vi "LVDimInterface.release.vi"(5 "error in (no error)":errorcluster) -> (19 "error out":errorcluster)   [LabVIEW 2013, in "LVDimInterface.lvlib"]
doc: "Releases (unlocks) the LVDimInterface after changes. This routine is intended for internal purposes only.\n\nLicense Agreement for this software:\n\nCopyright (C)\nGesellschaft für Schwerionenforschung, GSI\nPlanckstr. 1\n64291 Darmstadt\nGermany\n\nContact: D.Beck@gsi.de \n\nThis program is free software; you can redistribute it and/or modify it under the terms of the GNU General Public License as published by the Free Software Foundation; either version 2 of the license, or (at your option) any later version.\n\nThis program is distributed in the hope that it will be useful, but WITHOUT ANY WARRANTY; without even the implied warranty of MERCHANTABILITY or FITNESS FOR A PARTICULAR PURPOSE. See the GNU General License for more details (http://www.gnu.org).\n\nGesellschaft für Schwerionenforschung, GSI\nPlanckstr. 1, 64291 Darmstadt, Germany\nFor all questions and ideas contact: M.Richter@gsi.de, H.Brand@gsi.de or D.Beck@gsi.de.\nLast update: 17-JUN-2004"
uses:
  LVDimInterface.lvlib
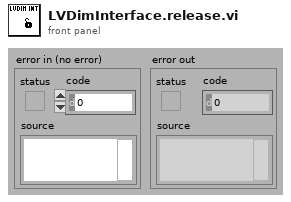
[diagram p1: front panel]
types:
  T1 = enum16{"unknown", "createSemaphore", "destroySemaphore", "getSemaphore"}
  T2 = typedef "Semaphore RefNum" = refnum<k1>
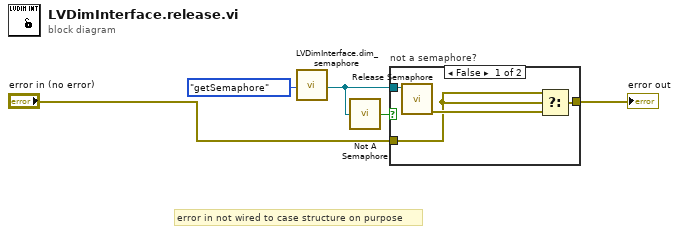
[diagram p0: block diagram]
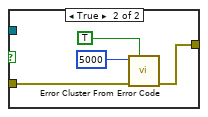
[diagram p2: hidden frame]
diagram:
  # "error in not wired to case structure on purpose"
  n1 = call "LVDimInterface.dim_semaphore.vi"("Action"=T1."getSemaphore") -> ("semaphore"=w2:T2)  [unwired: 18 in]
  n2 = call <vilib>:"Not A Semaphore.vi"("semaphore"=w2) -> ("not a semaphore"=w3:bool)
  n3 = case "not a semaphore?" shown="False" w3 {
    tunnel: [w9 w12] -> w5
    tunnel: "error in (no error)" -> [w7 w13]
    tunnel: w2 -> [w6 _]
    frame False {
      n4 = call <vilib>:"Release Semaphore.vi"("semaphore"=w6) -> ("error out"=w8:errorcluster)  [unwired: 5 in, 1 out]
      n5 = Select(t=w7, s=w7, f=w8) -> (s? t:f=w9:errorcluster)
    }
    frame True {
      n6 = call <vilib>:"Error Cluster From Error Code.vi"("show call chain? (False)"=TRUE ("status"), "error in (no error)"=w13, "error code (0)"=5000 ("code")) -> ("error out"=w12:errorcluster)  [unwired: 6 in]
    }
  }
  "error out" <- w5
